vi "práctica_32.vi"() -> ()   [LabVIEW 2019]
panel:
  in  "stop":bool
  out "Contraseña correcta":bool
  out "Pulsaciones":dbl
  in  "Contraseña":string
  in  "D":bool
  in  "C":bool
  in  "B":bool
  in  "A":bool
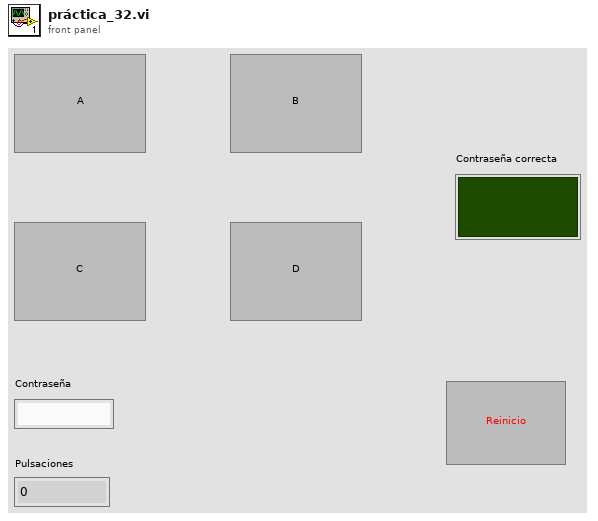
[diagram p1: front panel]
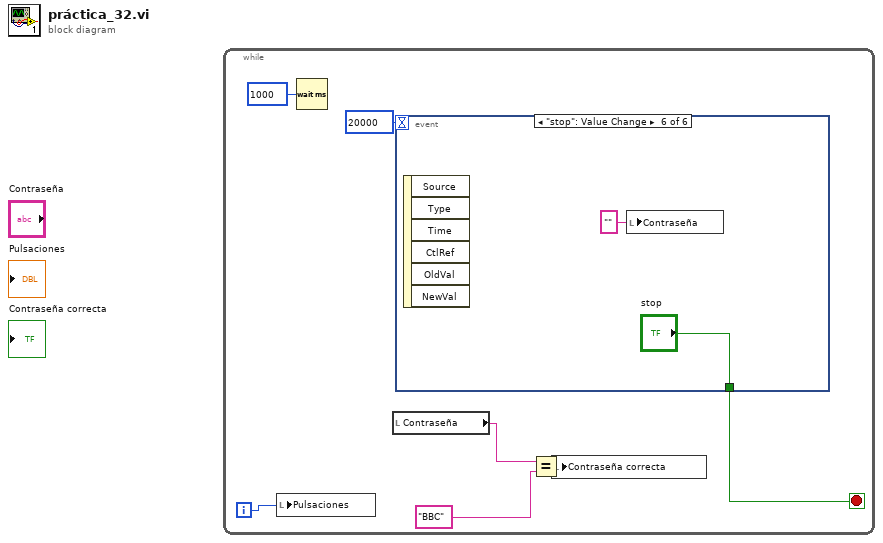
[diagram p0: block diagram]
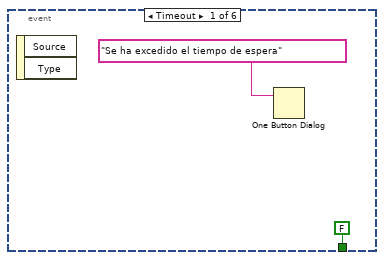
[diagram p2: hidden frame]
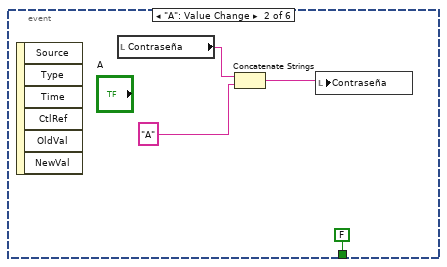
[diagram p3: hidden frame]
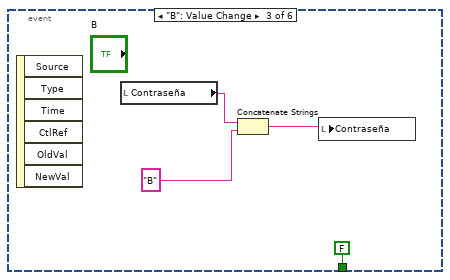
[diagram p4: hidden frame]
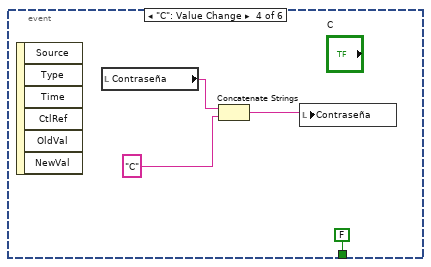
[diagram p5: hidden frame]
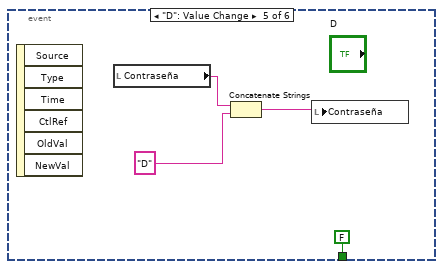
[diagram p6: hidden frame]
diagram:
  n1 = while {
    i -> [w6]
    stop <- w1 stop-if-true
    n2 = local write "Pulsaciones"(w6) -> ()
    n3 = Wait (ms)(milliseconds to wait=u32 1000) -> ()  [unwired: 1 out]
    n4 = local read "Contraseña"() -> (w2:string)
    n5 = event shown="[5] \"stop\": Value Change" {
      selector: _ -> [_ _ _ _ _ _]
      dyn-events: _ -> [_ _ _ _ _ _]
      timeout: 20000 -> [_ _ _ _ _ _]
      tunnel: [FALSE ("stop") FALSE ("stop") FALSE ("stop") FALSE ("stop") FALSE ("stop") "stop"] -> w1
      event Timeout {
        n6 = event-data() -> ()  [unwired: 1 in, 2 out]
        n7 = One Button Dialog(message="Se ha excedido el tiempo de espera") -> ()  [unwired: 1 in, 1 out]
      }
      event "A": Value Change {
        n8 = event-data() -> ()  [unwired: 1 in, 6 out]
        n9 = local read "Contraseña"() -> (w13:string)
        n10 = Concatenate Strings(w13, "A") -> (w11:string)
        n11 = local write "Contraseña"(w11) -> ()
      }
      event "B": Value Change {
        n12 = event-data() -> ()  [unwired: 1 in, 6 out]
        n13 = local read "Contraseña"() -> (w17:string)
        n14 = Concatenate Strings(w17, "B") -> (w15:string)
        n15 = local write "Contraseña"(w15) -> ()
      }
      event "C": Value Change {
        n16 = event-data() -> ()  [unwired: 1 in, 6 out]
        n17 = local read "Contraseña"() -> (w21:string)
        n18 = Concatenate Strings(w21, "C") -> (w19:string)
        n19 = local write "Contraseña"(w19) -> ()
      }
      event "D": Value Change {
        n20 = event-data() -> ()  [unwired: 1 in, 6 out]
        n21 = local read "Contraseña"() -> (w25:string)
        n22 = Concatenate Strings(w25, "D") -> (w24:string)
        n23 = local write "Contraseña"(w24) -> ()
      }
      event "stop": Value Change {
        n24 = event-data() -> ()  [unwired: 1 in, 6 out]
        n25 = local write "Contraseña"("" ("Contraseña")) -> ()
      }
    }
    n26 = Equal?(x=w2, y="BBC") -> (x = y?=w4:bool)
    n27 = local write "Contraseña correcta"(w4) -> ()
  }
